vi "test Future Can Timeout.vi"(8 "error in (no error)":errorcluster, 11 "TestCase in":refnum<class "Futures Tests.lvclass">) -> (0 "error out":errorcluster, 3 "TestCase out":refnum<class "Futures Tests.lvclass">)   [LabVIEW 2017, in "Futures Tests.lvclass"]
uses:
  Futures Tests.lvclass
  <vilib>/addons/_JKI Toolkits/VI Tester/TestCase.llb/TestCase.lvclass
  Futures/Futures.lvlib
  Futures/Future/Future.lvclass
  C:/Program Files (x86)/National Instruments/LabVIEW 2017/vi.lib/addons/_JKI Toolkits/VI Tester/TestCase.llb/TestCase.lvclass
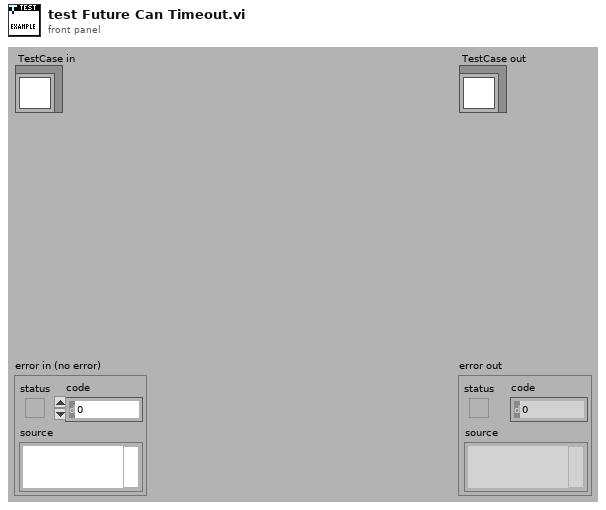
[diagram p1: front panel]
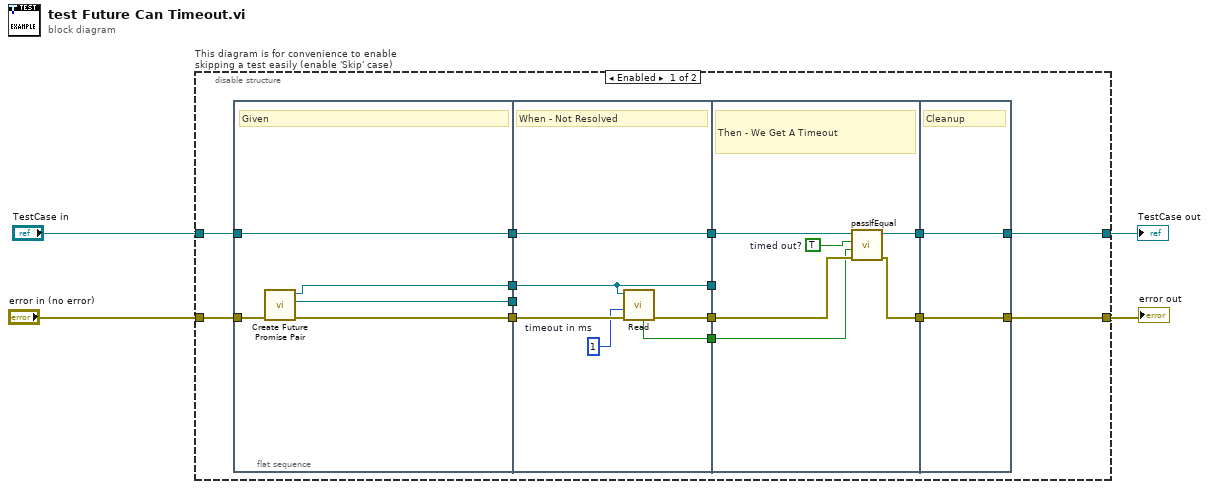
[diagram p0: block diagram]
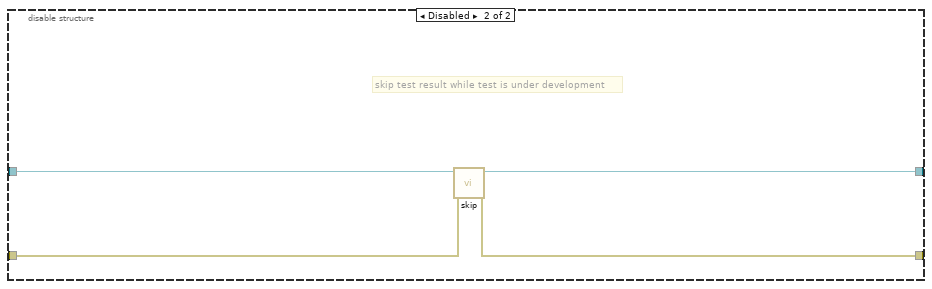
[diagram p2: hidden frame]
diagram:
  n1 = disable-structure "This diagram is for convenience to enable skipping a test easily (enable 'Skip' case)" shown="Enabled" {
    disable-tunnel: "TestCase in" -> [w12 w41]
    disable-tunnel: [w10 w39] -> w1
    disable-tunnel: [w9 w40] -> w3
    disable-tunnel: "error in (no error)" -> [w11 w38]
    frame Enabled {
      n2 = flat-sequence {
        tunnel: w11 -> [w22]
        tunnel: w12 -> [w23]
        tunnel: [w23] -> w18
        tunnel: [w21] -> w17
        tunnel: [w20] -> w8
        tunnel: [w19] -> w6
        tunnel: [w29] -> w16
        tunnel: [w27] -> w15
        tunnel: w18 -> [w29]
        tunnel: w17 -> [w26]
        tunnel: w8 -> [_]
        tunnel: [w28] -> w7
        tunnel: w6 -> [w28]
        tunnel: [w24] -> w5
        tunnel: [w34] -> w14
        tunnel: [w33] -> w13
        tunnel: w16 -> [w35]
        tunnel: w15 -> [w32]
        tunnel: w7 -> [_]
        tunnel: w5 -> [w31]
        tunnel: [w36] -> w9
        tunnel: [w37] -> w10
        tunnel: w14 -> [w37]
        tunnel: w13 -> [w36]
        frame #0 {
          # "Given"
          n3 = call "Create Future Promise Pair.vi"("error in (no error)"=w22) -> ("error out"=w21:errorcluster, "Promise out"=w20:refnum<class "Promise.lvclass">, "Future out"=w19:refnum<class "Future.lvclass">)  [unwired: 8 in]
        }
        frame #1 {
          w25 = 1  # timeout in ms
          # "When - Not Resolved"
          n4 = call "Read.vi"("error in (no error)"=w26, "timeout in ms (60 sec)"=w25, "Future in"=w28) -> ("error out"=w27:errorcluster, "timed out?"=w24:bool)  [unwired: 4 in, 3 out]
        }
        frame #2 {
          w30 = TRUE  # timed out?
          # "Then - We Get A Timeout"
          n5 = call-dynamic "passIfEqual.vi"("error in (no error)"=w32, "y"=w31, "x"=w30, "TestCase in"=w35) -> ("error out"=w33:errorcluster, "TestCase out"=w34:refnum<class "Futures Tests.lvclass">)  [unwired: 6 in]
        }
        frame #3 {
          # "Cleanup"
        }
      }
    }
    frame Disabled {
      # "skip test result while test is under development"
      n6 = call <vilib>:"skip.vi"("error in (no error)"=w38, "TestCase in"=w41) -> ("error out"=w40:errorcluster, "TestCase out"=w39:refnum<class "Futures Tests.lvclass">)  [unwired: 8 in]
    }
  }
  "error out" <- w3
  "TestCase out" <- w1
